vi "log analysis_gps.vi"() -> ()   [LabVIEW 2018] (continued)
113.233672\t8.086500\t-0.914034\t0.254354\t-14.267434\t0.261000\t-0.076000\n\t\n15:18:13.8\tlog_raw\tgps_raw\t#INSPVAXA,USB3,0,48.5,FINESTEERING,2107,281911.800,02000000,471d,15824;INS_ALIGNMENT_COMPLETE,INS_RTKFIXED,37.37115003469,126.72315448526,8.0928,22.3000,-0.0862,0.2747,0.0289,-0.974037724,0.304621853,104.802649899,0.4114,0.2983,0.5457,0.1097,0.0931,0.0770,0.1565,0.1577,4.9486,0f000001,0*2c2c9bcb\n\tsystem status\tnormal 2 28.100000 0 0\trobot status\t205.446896\t113.183810\t8.092800\t-0.974038\t0.304622\t-14.802650\t0.328000\t0.023000\n\t\n15:18:14.3\tlog_raw\tgps_raw\t\tsystem status\tnormal 2 28.100000 0 0\trobot status\t205.568847\t113.140219\t8.095700\t-0.943829\t0.162609\t-15.208872\t0.367000\t0.091000\n\t\n15:18:14.8\tlog_raw\tgps_raw\t\tsystem status\tnormal 2 28.100000 0 0\trobot status\t205.704066\t113.089880\t8.099100\t-0.874358\t-0.017169\t-15.670703\t0.260000\t-0.072000\n\t\n15:18:15.3\tlog_raw\tgps_raw\t\tsystem status\tnormal 2 28.100000 0 0\trobot status\t205.839267\t113.039134\t8.101800\t-0.860929\t-0.049716\t-16.043729\t0.318000\t0.015000\n\t\n15:18:15.8\tlog_raw\tgps_raw\t\tsystem status\tnormal 2 28.200000 0 0\trobot status\t205.974959\t112.988852\t8.103900\t-0.997845\t-0.009947\t-16.323608\t0.309000\t-0.001000\n\t\n15:18:16.3\tlog_raw\tgps_raw\t\tsystem status\tnormal 2 28.100000 0 0\trobot status\t206.103169\t112.938952\t8.105500\t-1.104598\t0.085353\t-16.584449\t0.300000\t-0.006000\n\t\n15:18:16.8\tlog_raw\tgps_raw\t\tsystem status\tnormal 2 28.100000 0 0\trobot status\t206.234047\t112.885788\t8.106200\t-1.056143\t0.296378\t-16.759396\t0.296000\t0.005000\n\t\n15:18:17.3\tlog_raw\tgps_raw\t\tsystem status\tnormal 2 28.100000 0 0\trobot status\t206.364780\t112.833450\t8.107500\t-1.030113\t0.365795\t-16.939127\t0.299000\t0.016000\n\t\n15:18:17.8\tlog_raw\tgps_raw\t\tsystem status\tnormal 2 28.100000 0 0\trobot status\t206.492890\t112.783184\t8.110300\t-1.134880\t0.359495\t-17.119683\t0.298000\t0.004000\n\t\n15:18:18.3\tlog_raw\tgps_raw\t#INSPVAXA,USB3,0,44.5,FINESTEERING,2107,281916.300,02000000,471d,15824;INS_ALIGNMENT_COMPLETE,INS_RTKFIXED,37.37114589383,126.72316794464,8.1130,22.3000,-0.1148,0.2616,0.0217,-1.148454264,0.358744068,107.173500933,0.4066,0.2960,0.5376,0.1089,0.0926,0.0764,0.1563,0.1575,4.9560,0f000001,0*04915923\n\tsystem status\tnormal 2 28.100000 0 0\trobot status\t206.639106\t112.724209\t8.113000\t-1.148454\t0.358744\t-17.173501\t0.299000\t0.014000\n\t\n15:18:18.8\tlog_raw\tgps_raw\t\tsystem status\tnormal 2 28.100000 0 0\trobot status\t206.763252\t112.674021\t8.115000\t-1.186823\t0.166172\t-17.276261\t0.302000\t0.017000\n\t\n15:18:19.3\tlog_raw\tgps_raw\t#INSPVAXA,USB3,0,45.5,FINESTEERING,2107,281917.300,02000000,471d,15824;INS_ALIGNMENT_COMPLETE,INS_RTKFIXED,37.37114488879,126.72317107328,8.1169,22.3000,-0.1215,0.2812,0.0224,-1.106333570,0.024690310,107.280249927,0.4087,0.2971,0.5398,0.1096,0.0930,0.0767,0.1563,0.1576,4.9575,0f000001,0*9d9688b2\n\tsystem status\tnormal 2 28.100000 0 0\trobot status\t206.916236\t112.612658\t8.116900\t-1.106334\t0.024690\t-17.280250\t0.247000\t0.103000\n\t\n15:18:19.8\tlog_raw\tgps_raw\t\tsystem status\tnormal 2 28.100000 0 0\trobot status\t207.042539\t112.563268\t8.119000\t-1.153156\t0.036383\t-17.324836\t0.359000\t-0.081000\n\t\n15:18:20.3\tlog_raw\tgps_raw\t\tsystem status\tnormal 2 28.100000 0 0\trobot status\t207.173934\t112.511452\t8.122900\t-1.261936\t0.129516\t-17.070571\t0.459000\t-0.218000\n\t\n15:18:20.8\tlog_raw\tgps_raw\t#INSPVAXA,USB3,0,48.5,FINESTEERING,2107,281918.800,02000000,471d,15824;INS_ALIGNMENT_COMPLETE,INS_RTKFIXED,37.37114346070,126.72317566723,8.1280,22.3000,-0.1055,0.2660,0.0189,-1.458385155,0.133384448,106.568583790,0.4097,0.2978,0.5415,0.1097,0.0931,0.0768,0.1562,0.1576,4.9589,0f000001,0*d5a698ac\n\tsystem status\tnormal 2 28.000000 0 0\trobot status\t207.323160\t112.454152\t8.128000\t-1.458385\t0.133384\t-16.568584\t0.311000\t0.002000\n\t\n15:18:21.3\tlog_raw\tgps_raw\t\tsystem status\tnormal 2 28.000000 0 0\trobot status\t207.444071\t112.408855\t8.130500\t-1.449095\t0.192120\t-16.048459\t0.246000\t0.096000\n\t\n15:18:21.8\tlog_raw\tgps_raw\t\tsystem status\tnormal 2 28.000000 0 0\trobot status\t207.576921\t112.362055\t8.132800\t-1.443864\t0.249922\t-15.418828\t0.394000\t-0.135000\n\t\n15:18:22.3\tlog_raw\tgps_raw\t\tsystem status\tnormal 2 27.900000 0 0\trobot status\t207.713267\t112.314966\t8.135200\t-1.432681\t0.160243\t-14.804981\t0.313000\t0.006000\n\t\n15:18:22.8\tlog_raw\tgps_raw\t#INSPVAXA,USB3,0,44.0,FINESTEERING,2107,281920.800,02000000,471d,15824;INS_ALIGNMENT_COMPLETE,INS_RTKFIXED,37.37114173890,126.72318175372,8.1382,22.3000,-0.1108,0.2593,0.0206,-1.441924072,0.214033238,104.164659813,0.4062,0.2959,0.5371,0.1088,0.0925,0.0764,0.1560,0.1575,4.9615,0f000001,0*96e1255f\n\tsystem status\tnormal 2 27.900000 0 0\trobot status\t207.862291\t112.263046\t8.138200\t-1.441924\t0.214033\t-14.164660\t0.280000\t0.030000\n\t\n15:18:23.3\tlog_raw\tgps_raw\t\tsystem status\tnormal 2 28.000000 0 0\trobot status\t207.983782\t112.223591\t8.140200\t-1.548397\t0.210381\t-13.589704\t0.258000\t0.062000\n\t\n15:18:23.8\tlog_raw\tgps_raw\t\tsystem status\tnormal 2 28.000000 0 0\trobot status\t208.119249\t112.180453\t8.141900\t-1.521400\t0.192125\t-13.096901\t0.307000\t-0.002000\n\t\n15:18:24.3\tlog_raw\tgps_raw\t\tsystem status\tnormal 2 28.000000 0 0\trobot status\t208.256790\t112.138571\t8.142800\t-1.453369\t0.256191\t-12.688055\t0.357000\t-0.086000\n\t\n15:18:24.8\tlog_raw\tgps_raw\t#INSPVAXA,USB3,0,48.0,FINESTEERING,2107,281922.800,02000000,471d,15824;INS_ALIGNMENT_COMPLETE,INS_RTKFIXED,37.37114021696,126.72318792765,8.1435,22.3000,-0.0885,0.2559,0.0232,-1.379339371,0.280141219,102.369247536,0.4099,0.2977,0.5413,0.1094,0.0930,0.0768,0.1560,0.1575,4.9637,0f000001,0*69df9f1e\n\tsystem status\tnormal 2 28.100000 0 0\trobot status\t208.409168\t112.094120\t8.143500\t-1.379339\t0.280141\t-12.369248\t0.323000\t-0.029000\n\t\n15:18:25.3\tlog_raw\tgps_raw\t\tsystem status\tnormal 2 28.100000 0 0\trobot status\t208.532591\t112.056371\t8.143200\t-1.130688\t0.148244\t-12.263747\t0.257000\t0.068000\n\t\n15:18:25.8\tlog_raw\tgps_raw\t#INSPVAXA,USB3,0,48.0,FINESTEERING,2107,281923.800,02000000,471d,15824;INS_ALIGNMENT_COMPLETE,INS_RTKFIXED,37.37113946532,126.72319101111,8.1415,22.3000,-0.0919,0.2757,0.0244,-1.061632800,0.175078722,102.246819670,0.4052,0.2954,0.5349,0.1085,0.0923,0.0763,0.1558,0.1574,4.9646,0f000001,0*a7ce5637\n\tsystem status\tnormal 2 28.100000 0 0\trobot status\t208.682296\t112.010693\t8.141500\t-1.061633\t0.175079\t-12.246820\t0.369000\t-0.100000\n\t\n15:18:26.3\tlog_raw\tgps_raw\t#INSPVAXA,USB3,0,47.5,FINESTEERING,2107,281924.300,02000000,471d,15824;INS_ALIGNMENT_COMPLETE,INS_RTKFIXED,37.37113911142,126.72319252846,8.1410,22.3000,-0.0952,0.2671,0.0232,-1.111033615,0.347415537,102.293993552,0.4024,0.2943,0.5302,0.1081,0.0921,0.0760,0.1558,0.1574,4.9658,0f000001,0*38544010\n\tsystem status\tnormal 2 28.100000 0 0\trobot status\t208.816700\t111.971412\t8.141000\t-1.111034\t0.347416\t-12.293994\t0.288000\t0.003000\n\t\n15:18:26.8\tlog_raw\tgps_raw\t\tsystem status\tnormal 2 28.100000 0 0\trobot status\t208.937676\t111.937072\t8.141200\t-1.176079\t0.471279\t-12.366041\t0.296000\t-0.021000\n\t\n15:18:27.3\tlog_raw\tgps_raw\t#INSPVAXA,USB3,0,45.0,FINESTEERING,2107,281925.300,02000000,471d,15824;INS_ALIGNMENT_COMPLETE,INS_RTKFIXED,37.37113840523,126.72319556014,8.1418,22.3000,-0.0995,0.2785,0.0107,-1.061115952,0.585903196,102.432927019,0.4060,0.2962,0.5334,0.1089,0.0927,0.0764,0.1559,0.1575,4.9673,0f000001,0*3a408327\n\tsystem status\tnormal 2 28.100000 0 0\trobot status\t209.085242\t111.893029\t8.141800\t-1.061116\t0.585903\t-12.432927\t0.300000\t-0.015000\n\t\n15:18:27.8\tlog_raw\tgps_raw\t\tsystem status\tnormal 2 28.100000 0 0\trobot status\t209.207574\t111.855880\t8.141900\t-1.051191\t0.670756\t-12.515029\t0.297000\t-0.021000\n\t\n15:18:28.3\tlog_raw\tgps_raw\t\tsystem status\tnormal 2 28.100000 0 0\trobot status\t209.344633\t111.814282\t8.142700\t-1.005218\t0.472311\t-12.681806\t0.294000\t-0.019000\n\t\n15:18:28.8\tlog_raw\tgps_raw\t#INSPVAXA,USB3,0,47.0,FINESTEERING,2107,281926.800,02000000,471d,15824;INS_ALIGNMENT_COMPLETE,INS_RTKFIXED,37.37113727918,126.72320023038,8.1455,22.3000,-0.1010,0.2911,0.0183,-0.984134489,0.435250920,102.983735265,0.4086,0.2974,0.5364,0.1094,0.0930,0.0766,0.1559,0.1575,4.9689,0f000001,0*added2fa\n\tsystem status\tnormal 2 28.100000 0 0\trobot status\t209.498924\t111.768044\t8.145500\t-0.984134\t0.435251\t-12.983735\t0.298000\t-0.026000\n\t\n15:18:29.3\tlog_raw\tgps_raw\t#INSPVAXA,USB3,0,47.0,FINESTEERING,2107,281927.300,02000000,471d,15824;INS_ALIGNMENT_COMPLETE,INS_RTKFIXED,37.37113689419,126.72320185554,8.1485,22.3000,-0.1162,0.2988,0.0149,-1.006289928,0.413812859,103.207528579,0.4104,0.2981,0.5392,0.1096,0.0931,0.0768,0.1559,0.1575,4.9705,0f000001,0*f16ca07f\n\tsystem status\tnormal 2 28.100000 0 0\trobot status\t209.642878\t111.725313\t8.148500\t-1.006290\t0.413813\t-13.207529\t0.300000\t-0.023000\n\t\n15:18:29.8\tlog_raw\tgps_raw\t\tsystem status\tnormal 2 28.100000 0 0\trobot status\t209.771603\t111.686476\t8.150800\t-1.004280\t0.360850\t-13.482463\t0.299000\t-0.023000\n\t\n15:18:30.3\tlog_raw\tgps_raw\t#INSPVAXA,USB3,0,48.5,FINESTEERING,2107,281928.300,02000000,471d,15824;INS_ALIGNMENT_COMPLETE,INS_RTKFIXED,37.37113611712,126.72320505771,8.1519,22.3000,-0.1090,0.2747,0.0204,-1.003980173,0.404401271,103.811290655,0.4113,0.2984,0.5414,0.1096,0.0931,0.0769,0.1559,0.1574,4.9721,0f000001,0*ce8a0efc\n\tsystem status\tnormal 2 28.100000 0 0\trobot status\t209.926521\t111.639063\t8.151900\t-1.003980\t0.404401\t-13.811291\t0.313000\t-0.013000\n\t\n15:18:30.8\tlog_raw\tgps_raw\t\tsystem status\tnormal 2 28.100000 0 0\trobot status\t210.050220\t111.601287\t8.152500\t-1.081434\t0.192161\t-14.259836\t0.314000\t-0.006000\n\t\n15:18:31.3\tlog_raw\tgps_raw\t#INSPVAXA,USB3,0,47.0,FINESTEERING,2107,281929.300,02000000,471d,15824;INS_ALIGNMENT_COMPLETE,INS_RTKFIXED,37.37113535023,126.72320815380,8.1534,22.3000,-0.0933,0.2709,0.0146,-1.164082323,0.102490422,104.875233542,0.4118,0.2986,0.5433,0.1096,0.0930,0.0770,0.1559,0.1574,4.9735,0f000001,0*94f0b5d4\n\tsystem status\tnormal 2 28.100000 0 0\trobot status\t210.200767\t111.553943\t8.153400\t-1.164082\t0.102490\t-14.875234\t0.369000\t0.072000\n\t\n15:18:31.8\tlog_raw\tgps_raw\t\tsystem status\tnormal 2 28.000000 0 0\trobot status\t210.323789\t111.513594\t8.154400\t-1.166935\t0.086527\t-15.447802\t0.352000\t0.056000\n\t\n15:18:32.3\tlog_raw\tgps_raw\t#INSPVAXA,USB3,0,49.0,FINESTEERING,2107,281930.300,02000000,471d,15824;INS_ALIGNMENT_COMPLETE,INS_RTKFIXED,37.37113452225,126.72321122959,8.1544,22.3000,-0.0922,0.2630,0.0022,-1.151432888,0.140260407,106.440387814,0.4107,0.2981,0.5430,0.1094,0.0928,0.0769,0.1559,0.1573,4.9747,0f000001,0*0b618f55\n\tsystem status\tnormal 2 28.000000 0 0\trobot status\t210.473216\t111.462043\t8.154400\t-1.151433\t0.140260\t-16.440388\t0.352000\t0.063000\n\t\n15:18:32.8\tlog_raw\tgps_raw\t\tsystem status\tnormal 2 28.000000 0 0\trobot status\t210.593839\t111.416960\t8.153900\t-1.009363\t0.310031\t-17.172659\t0.276000\t-0.068000\n\t\n15:18:33.3\tlog_raw\tgps_raw\t#INSPVAXA,USB3,0,46.5,FINESTEERING,2107,281931.300,02000000,471d,15824;INS_ALIGNMENT_COMPLETE,INS_RTKFIXED,37.37113361810,126.72321422448,8.1520,22.3000,-0.1052,0.2573,0.0056,-1.026339902,0.274196380,108.020288204,0.4094,0.2975,0.5419,0.1091,0.0927,0.0767,0.1558,0.1572,4.9758,0f000001,0*a4843e8d\n\tsystem status\tnormal 2 28.000000 0 0\trobot status\t210.738498\t111.361690\t8.152000\t-1.026340\t0.274196\t-18.020288\t0.280000\t-0.056000\n\t\n15:18:33.8\tlog_raw\tgps_raw\t#INSPVAXA,USB3,0,46.5,FINESTEERING,2107,281931.800,02000000,471d,15824;INS_ALIGNMENT_COMPLETE,INS_RTKFIXED,37.37113315554,126.72321571726,8.1497,22.3000,-0.1071,0.2546,0.0196,-1.189773358,0.228457398,108.723422614,0.4094,0.2975,0.5419,0.1091,0.0927,0.0767,0.1558,0.1572,4.9758,0f000001,0*2e0e4421\n\tsystem status\tnormal 2 28.000000 0 0\trobot status\t210.870726\t111.310349\t8.149700\t-1.189773\t0.228457\t-18.723423\t0.344000\t0.043000\n\t\n15:18:34.3\tlog_raw\tgps_raw\t\tsystem status\tnormal 2 28.000000 0 0\trobot status\t210.990843\t111.261950\t8.149000\t-1.145411\t0.022083\t-19.237081\t0.379000\t0.107000\n\t\n15:18:34.8\tlog_raw\tgps_raw\t#INSPVAXA,USB3,0,46.5,FINESTEERING,2107,281932.800,02000000,471d,15824;INS_ALIGNMENT_COMPLETE,INS_RTKFIXED,37.37113218049,126.72321869652,8.1511,22.3000,-0.1122,0.2507,0.0244,-0.970343448,0.146977674,109.553158017,0.4088,0.2971,0.5408,0.1090,0.0926,0.0766,0.1558,0.1571,4.9770,0f000001,0*3507ce24\n\tsystem status\tnormal 2 28.100000 0 0\trobot status\t211.134624\t111.202127\t8.151100\t-0.970343\t0.146978\t-19.553158\t0.277000\t-0.042000\n\t\n15:18:35.3\tlog_raw\tgps_raw\t#INSPVAXA,USB3,0,46.5,FINESTEERING,2107,281933.300,02000000,471d,15824;INS_ALIGNMENT_COMPLETE,INS_RTKFIXED,37.37113167702,126.72322018624,8.1496,22.3000,-0.1082,0.2476,0.0112,-0.825942181,0.095830764,109.777034035,0.4078,0.2967,0.5396,0.1089,0.0928,0.0765,0.1558,0.1571,4.9781,0f000001,0*1bc6ffe3\n\tsystem status\tnormal 2 28.100000 0 0\trobot status\t211.266581\t111.146246\t8.149600\t-0.825942\t0.095831\t-19.777034\t0.276000\t-0.027000\n\t\n15:18:35.8\tlog_raw\tgps_raw\t\tsystem status\tnormal 2 28.100000 0 0\trobot status\t211.383963\t111.097377\t8.147600\t-0.886599\t-0.030831\t-20.009787\t0.307000\t0.005000\n\t\n15:18:36.3\tlog_raw\tgps_raw\t\tsystem status\tnormal 2 28.100000 0 0\trobot status\t211.510009\t111.044758\t8.145100\t-0.938351\t-0.047781\t-20.227400\t0.297000\t0.000000\n\t\n15:18:36.8\tlog_raw\tgps_raw\t#INSPVAXA,USB3,0,48.5,FINESTEERING,2107,281934.800,02000000,471d,15824;INS_ALIGNMENT_COMPLETE,INS_RTKFIXED,37.37113025084,126.72322449049,8.1432,22.3000,-0.1047,0.2449,0.0092,-0.950644980,-0.057069061,110.390138086,0.4095,0.2975,0.5414,0.1094,0.0930,0.0767,0.1558,0.1572,4.9791,0f000001,0*563aefdc\n\tsystem status\tnormal 2 28.100000 0 0\trobot status\t211.647845\t110.987953\t8.143200\t-0.950645\t-0.057069\t-20.390138\t0.295000\t0.016000\n\t\n15:18:37.3\tlog_raw\tgps_raw\t#INSPVAXA,USB3,0,46.5,FINESTEERING,2107,281935.300,02000000,471d,15824;INS_ALIGNMENT_COMPLETE,INS_RTKFIXED,37.37112977302,126.72322590337,8.1419,22.3000,-0.1049,0.2498,0.0104,-0.942926672,-0.039965742,110.562621563,0.4110,0.2981,0.5430,0.1097,0.0932,0.0768,0.1557,0.1572,4.9802,0f000001,0*75823065\n\tsystem status\tnormal 2 28.100000 0 0\trobot status\t211.772995\t110.934919\t8.141900\t-0.942927\t-0.039966\t-20.562622\t0.303000\t0.015000\n\t\n15:18:37.8\tlog_raw\tgps_raw\t#INSPVAXA,USB3,0,46.5,FINESTEERING,2107,281935.800,02000000,471d,15824;INS_ALIGNMENT_COMPLETE,INS_RTKFIXED,37.37112927929,126.72322735116,8.1404,22.3000,-0.1170,0.2611,0.0107,-1.050315231,0.030356412,110.657182537,0.4110,0.2981,0.5430,0.1097,0.0932,0.0768,0.1557,0.1572,4.9802,0f000001,0*518b09cb\n\tsystem status\tnormal 2 28.100000 0 0\trobot status\t211.901238\t110.880119\t8.140400\t-1.050315\t0.030356\t-20.657183\t0.298000\t0.012000\n\t\n15:18:38.3\tlog_raw\tgps_raw\t\tsystem status\tnormal 2 28.100000 0 0\trobot status\t212.021991\t110.826901\t8.139400\t-1.016485\t0.243724\t-20.726094\t0.302000\t0.024000\n\t\n15:18:38.8\tlog_raw\tgps_raw\t#INSPVAXA,USB3,0,46.5,FINESTEERING,2107,281936.800,02000000,471d,15824;INS_ALIGNMENT_COMPLETE,INS_RTKFIXED,37.37112820521,126.72323038225,8.1394,22.3000,-0.1018,0.2637,0.0146,-1.057508289,0.307807352,110.761201411,0.4116,0.2984,0.5442,0.1099,0.0933,0.0768,0.1556,0.1572,4.9813,0f000001,0*af3d1803\n\tsystem status\tnormal 2 28.100000 0 0\trobot status\t212.169727\t110.760906\t8.139400\t-1.057508\t0.307807\t-20.761201\t0.298000\t0.009000\n\t\n15:18:39.3\tlog_raw\tgps_raw\t#INSPVAXA,USB3,0,50.5,FINESTEERING,2107,281937.300,02000000,471d,15824;INS_ALIGNMENT_COMPLETE,INS_RTKFIXED,37.37112766751,126.72323189029,8.1401,22.3000,-0.1026,0.2581,0.0148,-1.068160739,0.434910636,110.781904334,0.4120,0.2986,0.5450,0.1099,0.0934,0.0769,0.1555,0.1571,4.9826,0f000001,0*c1896a38\n\tsystem status\tnormal 2 28.100000 0 0\trobot status\t212.303307\t110.701226\t8.140100\t-1.068161\t0.434911\t-20.781904\t0.262000\t0.067000\n\t\n15:18:39.8\tlog_raw\tgps_raw\t#INSPVAXA,USB3,0,50.5,FINESTEERING,2107,281937.800,02000000,471d,15824;INS_ALIGNMENT_COMPLETE,INS_RTKFIXED,37.37112712976,126.72323340459,8.1402,22.3000,-0.1084,0.2649,0.0122,-1.080841395,0.445033455,110.675623077,0.4120,0.2986,0.5450,0.1099,0.0934,0.0769,0.1555,0.1571,4.9826,0f000001,0*491a3d94\n\tsystem status\tnormal 2 28.100000 0 0\trobot status\t212.437441\t110.641541\t8.140200\t-1.080841\t0.445033\t-20.675623\t0.304000\t0.016000\n\t\n15:18:40.3\tlog_raw\tgps_raw\t#INSPVAXA,USB3,0,48.0,FINESTEERING,2107,281938.300,02000000,471d,15824;INS_ALIGNMENT_COMPLETE,INS_RTKFIXED,37.37112660699,126.72323489042,8.1401,22.3000,-0.1000,0.2525,0.0063,-1.085397063,0.578788009,110.287744750,0.4123,0.2988,0.5457,0.1100,0.0934,0.0769,0.1554,0.1571,4.9841,0f000001,0*2d3bbc15\n\tsystem status\tnormal 2 28.100000 0 0\trobot status\t212.569053\t110.583518\t8.140100\t-1.085397\t0.578788\t-20.287745\t0.343000\t-0.046000\n\t\n15:18:40.8\tlog_raw\tgps_raw\t\tsystem status\tnormal 2 28.000000 0 0\trobot status\t212.688313\t110.532071\t8.140100\t-1.053466\t0.635759\t-19.821396\t0.389000\t-0.113000\n\t\n15:18:41.3\tlog_raw\tgps_raw\t#INSPVAXA,USB3,0,48.0,FINESTEERING,2107,281939.300,02000000,471d,15824;INS_ALIGNMENT_COMPLETE,INS_RTKFIXED,37.37112559001,126.72323792632,8.1403,22.3000,-0.1055,0.2758,-0.0006,-1.140987181,0.421010815,109.156991260,0.4088,0.2970,0.5408,0.1093,0.0930,0.0765,0.1552,0.1570,4.9858,0f000001,0*79dbeeff\n\tsystem status\tnormal 2 28.000000 0 0\trobot status\t212.837968\t110.470642\t8.140300\t-1.140987\t0.421011\t-19.156991\t0.464000\t-0.225000\n\t\n15:18:41.8\tlog_raw\tgps_raw\t#INSPVAXA,USB3,0,48.0,FINESTEERING,2107,281939.800,02000000,471d,15824;INS_ALIGNMENT_COMPLETE,INS_RTKFIXED,37.37112510387,126.72323945796,8.1419,22.3000,-0.1142,0.2830,0.0009,-1.038854179,0.260898620,108.398784803,0.4088,0.2970,0.5408,0.1093,0.0930,0.0765,0.1552,0.1570,4.9858,0f000001,0*5c0fede7\n\tsystem status\tnormal 2 27.900000 0 0\trobot status\t212.973639\t110.416685\t8.141900\t-1.038854\t0.260899\t-18.398785\t0.232000\t0.129000\n\t\n15:18:42.3\tlog_raw\tgps_raw\t\tsystem status\tnormal 2 27.800000 0 0\trobot status\t213.094310\t110.372130\t8.143700\t-1.147411\t0.248364\t-17.713610\t0.325000\t-0.023000\n\t\n15:18:42.8\tlog_raw\tgps_raw\t#INSPVAXA,USB3,0,46.0,FINESTEERING,2107,281940.800,02000000,471d,15824;INS_ALIGNMENT_COMPLETE,INS_RTKFIXED,37.37112421905,126.72324251509,8.1454,22.3000,-0.0917,0.2666,0.0165,-1.172718018,0.154583704,106.881501399,0.4059,0.2957,0.5358,0.1088,0.0926,0.0762,0.1550,0.1569,4.9872,0f000001,0*d9c0846d\n\tsystem status\tnormal 2 27.900000 0 0\trobot status\t213.244434\t110.318476\t8.145400\t-1.172718\t0.154584\t-16.881501\t0.323000\t-0.008000\n\t\n15:18:43.3\tlog_raw\tgps_raw\t#INSPVAXA,USB3,0,46.0,FINESTEERING,2107,281941.300,02000000,471d,15824;INS_ALIGNMENT_COMPLETE,INS_RTKFIXED,37.37112376695,126.72324410387,8.1465,22.3000,-0.0867,0.2640,0.0120,-1.227884261,0.058014022,106.288086050,0.4040,0.2951,0.5320,0.1086,0.0925,0.0760,0.1549,0.1568,4.9885,0f000001,0*dacbaea6\n\tsystem status\tnormal 2 27.900000 0 0\trobot status\t213.385166\t110.268297\t8.146500\t-1.227884\t0.058014\t-16.288086\t0.360000\t-0.080000\n\t\n15:18:43.8\tlog_raw\tgps_raw\t#INSPVAXA,USB3,0,46.0,FINESTEERING,2107,281941.800,02000000,471d,15824;INS_ALIGNMENT_COMPLETE,INS_RTKFIXED,37.37112332750,126.72324562221,8.1480,22.3000,-0.0872,0.2775,0.0087,-1.185427443,0.271965385,105.771989381,0.4040,0.2951,0.5320,0.1086,0.0925,0.0760,0.1549,0.1568,4.9885,0f000001,0*6fc02a4a\n\tsystem status\tnormal 2 28.000000 0 0\trobot status\t213.519658\t110.219521\t8.148000\t-1.185427\t0.271965\t-15.771989\t0.338000\t-0.036000\n\t\n15:18:44.3\tlog_raw\tgps_raw\t#INSPVAXA,USB3,0,48.0,FINESTEERING,2107,281942.300,02000000,471d,15824;INS_ALIGNMENT_COMPLETE,INS_RTKFIXED,37.37112291228,126.72324712545,8.1496,22.3000,-0.0882,0.2861,0.0099,-1.302160534,0.485080521,105.427907916,0.4030,0.2950,0.5294,0.1085,0.0925,0.0759,0.1549,0.1568,4.9897,0f000001,0*226a6453\n\tsystem status\tnormal 2 28.000000 0 0\trobot status\t213.652812\t110.173434\t8.149600\t-1.302161\t0.485081\t-15.427908\t0.406000\t-0.152000\n\t\n15:18:44.8\tlog_raw\tgps_raw\t#INSPVAXA,USB3,0,48.0,FINESTEERING,2107,281942.800,02000000,471d,15824;INS_ALIGNMENT_COMPLETE,INS_RTKFIXED,37.37112248759,126.72324869742,8.1506,22.3000,-0.0906,0.2829,0.0087,-1.416858091,0.320755573,105.114795692,0.4030,0.2950,0.5294,0.1085,0.0925,0.0759,0.1549,0.1568,4.9897,0f000001,0*d431e262\n\tsystem status\tnormal 2 28.000000 0 0\trobot status\t213.792055\t110.126297\t8.150600\t-1.416858\t0.320756\t-15.114796\t0.206000\t0.151000\n\t\n15:18:45.3\tlog_raw\tgps_raw\t#DUALANTENNAHEADINGA,USB3,0,49.0,FINESTEERING,2107,281943.300,02000000,d426,15824;SOL_COMPUTED,NARROW_FLOAT,-1.000000000,117.129844666,-65.553436279,0.0,360.000000000,180.000000000,\"631T\",17,7,7,7,04,00,20,03*a0d5c722\n\tsystem status\tnormal 2 28.000000 0 0\trobot status\t213.929277\t110.079751\t8.151600\t-1.442984\t0.403224\t-14.941741\t0.336000\t-0.059000\n\t\n15:18:45.8\tlog_raw\tgps_raw\t#INSPVAXA,USB3,0,49.0,FINESTEERING,2107,281943.800,02000000,471d,15824;INS_ALIGNMENT_COMPLETE,INS_RTKFIXED,37.37112165725,126.72325176425,8.1526,22.3000,-0.0982,0.2663,0.0142,-1.467433834,0.522949098,104.939300217,0.4063,0.2966,0.5325,0.1091,0.0930,0.0763,0.1549,0.1569,4.9906,0f000001,0*8fab3056\n\tsystem status\tnormal 2 28.100000 0 0\trobot status\t214.063710\t110.034135\t8.152600\t-1.467434\t0.522949\t-14.939300\t0.263000\t0.038000\n\t\n15:18:46.3\tlog_raw\tgps_raw\t#INSPVAXA,USB3,0,49.0,FINESTEERING,2107,281944.300,02000000,471d,15824;INS_ALIGNMENT_COMPLETE,INS_RTKFIXED,37.37112121835,126.72325329902,8.1549,22.3000,-0.0986,0.2706,0.0194,-1.288520157,0.440494920,104.991020886,0.4098,0.2978,0.5362,0.1096,0.0931,0.0766,0.1549,0.1570,4.9912,0f000001,0*9299408f\n\tsystem status\tnormal 2 28.100000 0 0\trobot status\t214.199657\t109.985420\t8.154900\t-1.288520\t0.440495\t-14.991021\t0.336000\t-0.064000\n\t\n15:18:46.8\tlog_raw\tgps_raw\t#INSPVAXA,USB3,0,49.0,FINESTEERING,2107,281944.800,02000000,471d,15824;INS_ALIGNMENT_COMPLETE,INS_RTKFIXED,37.37112078350,126.72325484675,8.1574,22.3000,-0.0973,0.2817,0.0195,-1.314361795,0.302961739,105.060294350,0.4098,0.2978,0.5362,0.1096,0.0931,0.0766,0.1549,0.1570,4.9912,0f000001,0*74de03e1\n\tsystem status\tnormal 2 28.100000 0 0\trobot status\t214.336752\t109.937155\t8.157400\t-1.314362\t0.302962\t-15.060294\t0.300000\t-0.007000\n\t\n15:18:47.3\tlog_raw\tgps_raw\t#INSPVAXA,USB3,0,50.5,FINESTEERING,2107,281945.300,02000000,471d,15824;INS_ALIGNMENT_COMPLETE,INS_RTKFIXED,37.37112035973,126.72325634532,8.1592,22.3000,-0.0947,0.2865,0.0177,-1.337666761,0.342742337,105.119539475,0.4078,0.2967,0.5345,0.1091,0.0927,0.0765,0.1549,0.1569,4.9918,0f000001,0*40c63c80\n\tsystem status\tnormal 2 28.100000 0 0\trobot status\t214.469493\t109.890120\t8.159200\t-1.337667\t0.342742\t-15.119539\t0.301000\t-0.004000\n\t\n15:18:47.8\tlog_raw\tgps_raw\t#DUALANTENNAHEADINGA,USB3,0,50.5,FINESTEERING,2107,281945.800,02000000,d426,15824;SOL_COMPUTED,NARROW_FLOAT,-1.000000000,110.210548401,-43.006103516,0.0,360.000000000,180.000000000,\"631T\",17,7,7,7,04,00,20,03*d65a3eb4\n\tsystem status\tnormal 2 28.100000 0 0\trobot status\t214.602489\t109.843444\t8.161100\t-1.466597\t0.319306\t-15.188465\t0.298000\t-0.016000\n\t\n15:18:48.3\tlog_raw\tgps_raw\t#DUALANTENNAHEADINGA,USB3,0,50.5,FINESTEERING,2107,281946.300,02000000,d426,15824;SOL_COMPUTED,NARROW_FLOAT,-1.000000000,136.716491699,-61.625274658,0.0,360.000000000,180.000000000,\"631T\",17,7,7,7,04,00,20,03*380a706b\n\tsystem status\tnormal 2 28.100000 0 0\trobot status\t214.739494\t109.795002\t8.162800\t-1.483580\t0.274543\t-15.266897\t0.302000\t-0.010000\n\t\n15:18:48.8\tlog_raw\tgps_raw\t#INSPVAXA,USB3,0,50.5,FINESTEERING,2107,281946.800,02000000,471d,15824;INS_ALIGNMENT_COMPLETE,INS_RTKFIXED,37.37111906801,126.72326090690,8.1646,22.3000,-0.0999,0.2885,0.0123,-1.416267608,0.329165481,105.354050291,0.4059,0.2956,0.5320,0.1087,0.0926,0.0762,0.1548,0.1568,4.9924,0f000001,0*28d47c8b\n\tsystem status\tnormal 2 28.100000 0 0\trobot status\t214.873551\t109.746748\t8.164600\t-1.416268\t0.329165\t-15.354050\t0.304000\t-0.010000\n\t\n15:18:49.3\tlog_raw\tgps_raw\t#INSPVAXA,USB3,0,45.5,FINESTEERING,2107,281947.300,02000000,471d,15824;INS_ALIGNMENT_COMPLETE,INS_RTKFIXED,37.37111863332,126.72326240814,8.1666,22.3000,-0.0961,0.2751,0.0203,-1.384816441,0.416422862,105.503918541,0.4041,0.2951,0.5298,0.1085,0.0924,0.0761,0.1549,0.1568,4.9930,0f000001,0*a10fe9f6\n\tsystem status\tnormal 2 28.100000 0 0\trobot status\t215.006528\t109.698501\t8.166600\t-1.384816\t0.416423\t-15.503919\t0.295000\t-0.019000\n\t\n15:18:49.8\tlog_raw\tgps_raw\t#INSPVAXA,USB3,0,45.5,FINESTEERING,2107,281947.800,02000000,471d,15824;INS_ALIGNMENT_COMPLETE,INS_RTKFIXED,37.37111818250,126.72326395318,8.1681,22.3000,-0.0954,0.2801,0.0190,-1.275593165,0.401297013,105.699844035,0.4041,0.2951,0.5298,0.1085,0.0924,0.0761,0.1549,0.1568,4.9930,0f000001,0*107534c5\n\tsystem status\tnormal 2 28.100000 0 0\trobot status\t215.143385\t109.648463\t8.168100\t-1.275593\t0.401297\t-15.699844\t0.297000\t-0.014000\n\t\n15:18:50.3\tlog_raw\tgps_raw\t#INSPVAXA,USB3,0,45.5,FINESTEERING,2107,281948.300,02000000,471d,15824;INS_ALIGNMENT_COMPLETE,INS_RTKFIXED,37.37111773045,126.72326549713,8.1704,22.3000,-0.0978,0.2931,0.0097,-1.304299318,0.393717319,105.933712093,0.4025,0.2945,0.5274,0.1083,0.0923,0.0760,0.1549,0.1567,4.9937,0f000001,0*f7f3e128\n\tsystem status\tnormal 2 28.100000 0 0\trobot status\t215.280146\t109.598289\t8.170400\t-1.304299\t0.393717\t-15.933712\t0.297000\t-0.013000\n\t\n15:18:50.8\tlog_raw\tgps_raw\t#DUALANTENNAHEADINGA,USB3,0,45.5,FINESTEERING,2107,281948.800,02000000,d426,15824;SOL_COMPUTED,NARROW_FLOAT,-1.000000000,181.763427734,-33.084808350,0.0,210.189346313,180.000000000,\"631T\",18,7,7,7,04,00,20,03*dd4d4ec1\n\tsystem status\tnormal 2 28.100000 0 0\trobot status\t215.414073\t109.546876\t8.173600\t-1.222613\t0.389782\t-16.150342\t0.298000\t-0.011000\n\t\n15:18:51.3\tlog_raw\tgps_raw\t#INSPVAXA,USB3,0,49.0,FINESTEERING,2107,281949.300,02000000,471d,15824;INS_ALIGNMENT_COMPLETE,INS_RTKFIXED,37.37111680262,126.72326852511,8.1763,22.3000,-0.0970,0.2807,0.0172,-1.183781176,0.416069138,106.325153596,0.4018,0.2942,0.5256,0.1083,0.0923,0.0759,0.1549,0.1566,4.9947,0f000001,0*47cb080a\n\tsystem status\tnormal 2 28.100000 0 0\trobot status\t215.548359\t109.495308\t8.176300\t-1.183781\t0.416069\t-16.325154\t0.298000\t-0.008000\n\t\n15:18:51.8\tlog_raw\tgps_raw\t#INSPVAXA,USB3,0,49.0,FINESTEERING,2107,281949.800,02000000,471d,15824;INS_ALIGNMENT_COMPLETE,INS_RTKFIXED,37.37111632001,126.72327008687,8.1784,22.3000,-0.0963,0.2886,0.0125,-1.143678600,0.359831061,106.512743553,0.4018,0.2942,0.5256,0.1083,0.0923,0.0759,0.1549,0.1566,4.9947,0f000001,0*07f750f1\n\tsystem status\tnormal 2 28.100000 0 0\trobot status\t215.686697\t109.441742\t8.178400\t-1.143679\t0.359831\t-16.512744\t0.302000\t-0.013000\n\t\n15:18:52.3\tlog_raw\tgps_raw\t#INSPVAXA,USB3,0,50.0,FINESTEERING,2107,281950.300,02000000,471d,15824;INS_ALIGNMENT_COMPLETE,INS_RTKFIXED,37.37111586312,126.72327158284,8.1822,22.3000,-0.0965,0.2844,0.0140,-1.158757889,0.473761966,106.723274256,0.4019,0.2945,0.5251,0.1083,0.0924,0.0759,0.1549,0.1566,4.9959,0f000001,0*c4604f56\n\tsystem status\tnormal 2 28.100000 0 0\trobot status\t215.819208\t109.391031\t8.182200\t-1.158758\t0.473762\t-16.723274\t0.298000\t-0.003000\n\t\n15:18:52.8\tlog_raw\tgps_raw\t#INSPVAXA,USB3,0,50.0,FINESTEERING,2107,281950.800,02000000,471d,15824;INS_ALIGNMENT_COMPLETE,INS_RTKFIXED,37.37111539537,126.72327311489,8.1870,22.3000,-0.0882,0.2799,0.0131,-1.063577950,0.631384742,106.921378709,0.4019,0.2945,0.5251,0.1083,0.0924,0.0759,0.1549,0.1566,4.9959,0f000001,0*182037fa\n\tsystem status\tnormal 2 28.100000 0 0\trobot status\t215.954914\t109.339114\t8.187000\t-1.063578\t0.631385\t-16.921379\t0.298000\t-0.001000\n\t\n15:18:53.3\tlog_raw\tgps_raw\t#DUALANTENNAHEADINGA,USB3,0,50.0,FINESTEERING,2107,281951.300,02000000,d426,15824;SOL_COMPUTED,NARROW_FLOAT,-1.000000000,139.470138550,7.252925396,0.0,360.000000000,180.000000000,\"631T\",16,7,7,7,04,00,20,03*6d09da6c\n\tsystem status\tnormal 2 28.100000 0 0\trobot status\t216.089759\t109.288189\t8.191800\t-1.034839\t0.729542\t-17.118886\t0.298000\t0.000000\n\t\n15:18:53.8\tlog_raw\tgps_raw\t#INSPVAXA,USB3,0,50.0,FINESTEERING,2107,281951.800,02000000,471d,15824;INS_ALIGNMENT_COMPLETE,INS_RTKFIXED,37.37111448325,126.72327615215,8.1961,22.3000,-0.0961,0.2823,0.0155,-1.049815385,0.768292718,107.282719412,0.4015,0.2942,0.5235,0.1082,0.0922,0.0758,0.1549,0.1565,4.9974,0f000001,0*bdafe358\n\tsystem status\tnormal 2 28.100000 0 0\trobot status\t216.223950\t109.237876\t8.196100\t-1.049815\t0.768293\t-17.282719\t0.298000\t-0.003000\n\t\n15:18:54.3\tlog_raw\tgps_raw\t#INSPVAXA,USB3,0,49.0,FINESTEERING,2107,281952.300,02000000,471d,15824;INS_ALIGNMENT_COMPLETE,INS_RTKFIXED,37.37111402480,126.72327764482,8.2001,22.3000,-0.0943,0.2854,0.0221,-1.074547440,0.687119581,107.404842007,0.4042,0.2955,0.5263,0.1087,0.0925,0.0761,0.1549,0.1565,4.9990,0f000001,0*5102a955\n\tsystem status\tnormal 2 28.100000 0 0\trobot status\t216.356168\t109.186991\t8.200100\t-1.074547\t0.687120\t-17.404842\t0.300000\t-0.002000\n\t\n15:18:54.8\tlog_raw\tgps_raw\t#INSPVAXA,USB3,0,49.0,FINESTEERING,2107,281952.800,02000000,471d,15824;INS_ALIGNMENT_COMPLETE,INS_RTKFIXED,37.37111356857,126.72327910492,8.2050,22.3000,-0.0959,0.2790,0.0249,-1.146713469,0.626149533,107.488269865,0.4042,0.2955,0.5263,0.1087,0.0925,0.0761,0.1549,0.1565,4.9990,0f000001,0*a4159e63\n\tsystem status\tnormal 2 28.100000 0 0\trobot status\t216.485501\t109.136354\t8.205000\t-1.146713\t0.626150\t-17.488270\t0.296000\t0.004000\n\t\n15:18:55.3\tlog_raw\tgps_raw\t#DUALANTENNAHEADINGA,USB3,0,51.5,FINESTEERING,2107,281953.300,02000000,d426,15824;SOL_COMPUTED,NARROW_FLOAT,-1.000000000,139.308395386,-63.930755615,0.0,360.000000000,171.725708008,\"631T\",19,7,7,7,04,00,20,03*aebc5255\n\tsystem status\tnormal 2 28.100000 0 0\trobot status\t216.619816\t109.082959\t8.208200\t-1.170202\t0.531585\t-17.534688\t0.298000\t0.004000\n\t\n15:18:55.8\tlog_raw\tgps_raw\t#DUALANTENNAHEADINGA,USB3,0,51.5,FINESTEERING,2107,281953.800,02000000,d426,15824;SOL_COMPUTED,NARROW_FLOAT,-1.000000000,139.742797852,-63.902252197,0.0,360.000000000,171.789428711,\"631T\",17,7,7,7,04,00,20,03*2ba0ac3f\n\tsystem status\tnormal 2 28.100000 0 0\trobot status\t216.757513\t109.028324\t8.209200\t-1.227407\t0.450832\t-17.644635\t0.305000\t0.003000\n\t\n15:18:56.3\tlog_raw\tgps_raw\t#INSPVAXA,USB3,0,49.5,FINESTEERING,2107,281954.300,02000000,471d,15824;INS_ALIGNMENT_COMPLETE,INS_RTKFIXED,37.37111212186,126.72328367661,8.2114,22.3000,-0.1061,0.2807,0.0084,-1.239615832,0.473328894,107.695107269,0.4028,0.2947,0.5241,0.1082,0.0921,0.0759,0.1549,0.1563,5.0021,0f000001,0*b68b8e11\n\tsystem status\tnormal 2 28.100000 0 0\trobot status\t216.890454\t108.975781\t8.211400\t-1.239616\t0.473329\t-17.695107\t0.307000\t0.003000\n\t\n15:18:56.8\tlog_raw\tgps_raw\t#DUALANTENNAHEADINGA,USB3,0,49.5,FINESTEERING,2107,281954.800,02000000,d426,15824;SOL_COMPUTED,NARROW_FLOAT,-1.000000000,123.390388489,-57.995361328,0.0,360.000000000,180.000000000,\"631T\",16,7,7,7,04,00,20,03*cd5e4259\n\tsystem status\tnormal 2 28.100000 0 0\trobot status\t217.023760\t108.923099\t8.214600\t-1.173148\t0.452181\t-17.734751\t0.304000\t0.001000\n\t\n15:18:57.3\tlog_raw\tgps_raw\t#DUALANTENNAHEADINGA,USB3,0,47.0,FINESTEERING,2107,281955.300,02000000,d426,15824;SOL_COMPUTED,NARROW_FLOAT,-1.000000000,132.237213135,-56.367187500,0.0,360.000000000,180.000000000,\"631T\",16,7,7,7,04,00,20,03*7928331b\n\tsystem status\tnormal 2 28.100000 0 0\trobot status\t217.160159\t108.869352\t8.216300\t-1.205497\t0.300570\t-17.770446\t0.271000\t0.059000\n\t\n15:18:57.8\tlog_raw\tgps_raw\t#DUALANTENNAHEADINGA,USB3,0,47.0,FINESTEERING,2107,281955.800,02000000,d426,15824;SOL_COMPUTED,NARROW_FLOAT,-1.000000000,131.490509033,-56.782928467,0.0,360.000000000,180.000000000,\"631T\",17,7,7,7,04,00,20,03*bed209ba\n\tsystem status\tnormal 2 28.100000 0 0\trobot status\t217.291693\t108.816650\t8.217000\t-1.220338\t0.256338\t-17.663149\t0.354000\t-0.086000\n\t\n15:18:58.3\tlog_raw\tgps_raw\t#DUALANTENNAHEADINGA,USB3,0,47.0,FINESTEERING,2107,281956.300,02000000,d426,15824;SOL_COMPUTED,NARROW_FLOAT,-1.000000000,120.002708435,27.323427200,0.0,360.000000000,180.000000000,\"631T\",18,7,7,7,04,00,20,03*7e70b057\n\tsystem status\tnormal 2 28.100000 0 0\trobot status\t217.421296\t108.765656\t8.217300\t-1.285586\t0.194299\t-17.466672\t0.307000\t-0.005000\n\t\n15:18:58.8\tlog_raw\tgps_raw\t#INSPVAXA,USB3,0,47.0,FINESTEERING,2107,281956.800,02000000,471d,15824;INS_ALIGNMENT_COMPLETE,INS_RTKFIXED,37.37110977016,126.72329115727,8.2173,22.3000,-0.1059,0.2673,0.0082,-1.256961721,0.075845968,107.131843549,0.4006,0.2939,0.5214,0.1078,0.0919,0.0757,0.1548,0.1562,5.0048,0f000001,0*c3de906c\n\tsystem status\tnormal 2 28.100000 0 0\trobot status\t217.553079\t108.714761\t8.217300\t-1.256962\t0.075846\t-17.131844\t0.277000\t0.040000\n\t\n15:18:59.3\tlog_raw\tgps_raw\t#INSPVAXA,USB3,0,49.0,FINESTEERING,2107,281957.300,02008000,471d,15824;INS_ALIGNMENT_COMPLETE,INS_RTKFIXED,37.37110932178,126.72329265930,8.2173,22.3000,-0.1030,0.2706,0.0074,-1.272872936,0.072348347,106.750132091,0.4007,0.2939,0.5208,0.1079,0.0919,0.0757,0.1548,0.1562,5.0062,0f000001,0*240beb48\n\tsystem status\tnormal 2 28.000000 0 0\trobot status\t217.686126\t108.664994\t8.217300\t-1.272873\t0.072348\t-16.750132\t0.291000\t0.011000\n\t\n15:18:59.8\tlog_raw\tgps_raw\t#DUALANTENNAHEADINGA,USB3,0,49.0,FINESTEERING,2107,281957.800,02008000,d426,15824;SOL_COMPUTED,NARROW_FLOAT,-1.000000000,114.580795288,38.922153473,0.0,360.000000000,180.000000000,\"631T\",20,7,7,7,04,00,20,03*611330d6\n\tsystem status\tnormal 2 28.000000 0 0\trobot status\t217.818289\t108.616774\t8.216900\t-1.286461\t0.054129\t-16.361997\t0.351000\t-0.055000\n\t\n15:19:00.3\tlog_raw\tgps_raw\t#DUALANTENNAHEADINGA,USB3,0,49.5,FINESTEERING,2107,281958.300,02008000,d426,15824;SOL_COMPUTED,NARROW_FLOAT,-1.000000000,104.400451660,-50.100708008,0.0,360.000000000,180.000000000,\"631T\",21,7,7,7,04,00,20,03*9c19a85a\n\tsystem status\tnormal 2 28.000000 0 0\trobot status\t217.951125\t108.569510\t8.215800\t-1.297113\t-0.037217\t-15.903945\t0.317000\t-0.015000\n\t\n15:19:00.8\tlog_raw\tgps_raw\t#DUALANTENNAHEADINGA,USB3,0,49.5,FINESTEERING,2107,281958.800,02008000,d426,15824;SOL_COMPUTED,NARROW_FLOAT,-1.000000000,106.192443848,-50.461669922,0.0,360.000000000,180.000000000,\"631T\",18,7,7,7,04,00,20,03*bd2737c2\n\tsystem status\tnormal 2 28.000000 0 0\trobot status\t218.085295\t108.523364\t8.214100\t-1.298690\t0.101611\t-15.423625\t0.264000\t0.060000\n\t\n15:19:01.3\tlog_raw\tgps_raw\t#DUALANTENNAHEADINGA,USB3,0,47.5,FINESTEERING,2107,281959.300,02008000,d426,15824;SOL_COMPUTED,NARROW_FLOAT,-1.000000000,102.626930237,-53.845886230,0.0,360.000000000,180.000000000,\"631T\",18,7,7,7,04,00,20,03*cccf90f6\n\tsystem status\tnormal 2 28.000000 0 0\trobot status\t218.218174\t108.479230\t8.213300\t-1.348834\t0.170230\t-14.989217\t0.288000\t0.030000\n\t\n15:19:01.8\tlog_raw\tgps_raw\t#DUALANTENNAHEADINGA,USB3,0,47.5,FINESTEERING,2107,281959.800,02008000,d426,15824;SOL_COMPUTED,NARROW_FLOAT,-1.000000000,103.518684387,-53.796081543,0.0,360.000000000,180.000000000,\"631T\",18,7,7,7,04,00,20,03*ff7adfc7\n\tsystem status\tnormal 2 28.000000 0 0\trobot status\t218.352131\t108.437190\t8.212200\t-1.540899\t0.247385\t-14.602198\t0.274000\t0.059000\n\t\n15:19:02.3\tlog_raw\tgps_raw\t#INSPVAXA,USB3,0,50.0,FINESTEERING,2107,281960.300,02008000,471d,15824;INS_ALIGNMENT_COMPLETE,INS_RTKFIXED,37.37110689498,126.72330172800,8.2108,22.3000,-0.0740,0.2831,-0.0019,-1.608231411,0.368287071,104.214278774,0.4044,0.2959,0.5251,0.1086,0.0926,0.0761,0.1548,0.1563,5.0100,0f000001,0*1846b4aa\n\tsystem status\tnormal 2 28.000000 0 0\trobot status\t218.489417\t108.395636\t8.210800\t-1.608231\t0.368287\t-14.214279\t0.433000\t-0.182000\n\t\n15:19:02.8\tlog_raw\tgps_raw\t#INSPVAXA,USB3,0,50.0,FINESTEERING,2107,281960.800,02008000,471d,15824;INS_ALIGNMENT_COMPLETE,INS_RTKFIXED,37.37110653498,126.72330326832,8.2098,22.3000,-0.0639,0.2787,-0.0006,-1.592412104,0.419958697,103.937219008,0.4044,0.2959,0.5251,0.1086,0.0926,0.0761,0.1548,0.1563,5.0100,0f000001,0*83162285\n\tsystem status\tnormal 2 28.000000 0 0\trobot status\t218.625856\t108.355678\t8.209800\t-1.592412\t0.419959\t-13.937219\t0.273000\t0.053000\n\t\n15:19:03.3\tlog_raw\tgps_raw\t#DUALANTENNAHEADINGA,USB3,0,46.5,FINESTEERING,2107,281961.300,02000000,d426,15824;SOL_COMPUTED,NARROW_FLOAT,-1.000000000,70.830032349,48.509868622,0.0,212.044555664,180.000000000,\"631T\",22,7,7,7,04,00,20,03*23813865\n\tsystem status\tnormal 2 28.100000 0 0\trobot status\t218.762630\t108.315447\t8.209500\t-1.566693\t0.295596\t-13.783376\t0.363000\t-0.090000\n\t\n15:19:03.8\tlog_raw\tgps_raw\t#DUALANTENNAHEADINGA,USB3,0,46.5,FINESTEERING,2107,281961.800,02000000,d426,15824;SOL_COMPUTED,NARROW_FLOAT,-1.000000000,72.091743469,46.579227448,0.0,218.795516968,180.000000000,\"631T\",20,7,7,7,04,00,20,03*2a3a9c35\n\tsystem status\tnormal 2 28.100000 0 0\trobot status\t218.900561\t108.274293\t8.209200\t-1.533585\t0.166784\t-13.693938\t0.262000\t0.064000\n\t\n15:19:04.3\tlog_raw\tgps_raw\t#DUALANTENNAHEADINGA,USB3,0,46.5,FINESTEERING,2107,281962.300,02000000,d426,15824;SOL_COMPUTED,NARROW_FLOAT,-1.000000000,79.598190308,38.491451263,0.0,329.037414551,180.000000000,\"631T\",18,7,7,7,04,00,20,03*3c555fcd\n\tsystem status\tnormal 2 28.100000 0 0\trobot status\t219.038780\t108.231931\t8.209000\t-1.526757\t0.262649\t-13.697319\t0.292000\t0.014000\n\t\n15:19:04.8\tlog_raw\tgps_raw\t#DUALANTENNAHEADINGA,USB3,0,46.5,FINESTEERING,2107,281962.800,02000000,d426,15824;SOL_COMPUTED,NARROW_FLOAT,-1.000000000,80.204544067,39.740882874,0.0,333.658050537,180.000000000,\"631T\",20,7,7,7,04,00,20,03*9ccf4ae9\n\tsystem status\tnormal 2 28.100000 0 0\trobot status\t219.176171\t108.188223\t8.208200\t-1.552273\t0.201310\t-13.772970\t0.304000\t-0.009000\n\t\n15:19:05.3\tlog_raw\tgps_raw\t#DUALANTENNAHEADINGA,USB3,0,45.5,FINESTEERING,2107,281963.300,02000000,d426,15824;SOL_COMPUTED,NARROW_FLOAT,-1.000000000,98.344001770,31.903175354,0.0,360.000000000,180.000000000,\"631T\",20,7,7,7,04,00,20,03*850b3b79\n\tsystem status\tnormal 2 28.100000 0 0\trobot status\t219.305773\t108.146770\t8.207700\t-1.593152\t0.025460\t-13.730583\t0.069000\t-0.015000\n\t\n15:19:05.8\tlog_raw\tgps_raw\t#DUALANTENNAHEADINGA,USB3,0,45.5,FINESTEERING,2107,281963.800,02000000,d426,15824;SOL_COMPUTED,NARROW_FLOAT,-1.000000000,99.070640564,30.000068665,0.0,360.000000000,180.000000000,\"631T\",18,7,7,7,04,00,20,03*27e895e1\n\tsystem status\tnormal 2 28.200000 0 0\trobot status\t219.295965\t108.139409\t8.206600\t-1.552409\t0.094425\t-13.844782\t-0.008000\t0.013000\n\t\n15:19:06.3\tlog_raw\tgps_raw\t#DUALANTENNAHEADINGA,USB3,0,47.5,FINESTEERING,2107,281964.300,02008000,d426,15824;SOL_COMPUTED,L1_FLOAT,-1.000000000,124.915382385,72.187736511,0.0,360.000000000,180.000000000,\"631T\",18,7,7,7,04,00,20,02*ef46fcdf\n\tsystem status\tnormal 2 28.200000 0 0\trobot status\t219.301691\t108.129830\t8.205900\t-1.561134\t0.086948\t-13.873180\t0.000000\t0.000000\n\t\n15:19:06.8\tlog_raw\tgps_raw\t#DUALANTENNAHEADINGA,USB3,0,47.5,FINESTEERING,2107,281964.800,02008000,d426,15824;SOL_COMPUTED,L1_FLOAT,-1.000000000,123.601234436,72.153076172,0.0,360.000000000,180.000000000,\"631T\",20,7,7,7,04,00,20,03*2f9fd869\n\tsystem status\tnormal 2 28.200000 0 0\trobot status\t219.300696\t108.122819\t8.205600\t-1.555405\t0.091635\t-13.868275\t0.000000\t0.000000\n\t\n15:19:07.3\tlog_raw\tgps_raw\t#DUALANTENNAHEADINGA,USB3,0,49.0,FINESTEERING,2107,281965.300,02008000,d426,15824;SOL_COMPUTED,NARROW_FLOAT,-1.000000000,138.902404785,50.477355957,0.0,360.000000000,180.000000000,\"631T\",21,7,7,7,04,00,20,
